vi "Filter Out Combined Source.vi"(1 "Sources In":T1[](array[typedef])) -> (0 "Sources Out":T1[](array[typedef]))   [LabVIEW 2009]
uses:
  Global Data/Transactions/Dataset Source.ctl
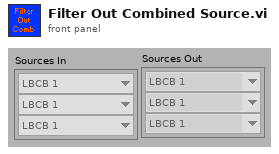
[diagram p1: front panel]
types:
  T1 = typedef "Dataset Source.ctl" = enum16{"LBCB 1", "LBCB 2", "Combined", "External Sensors"}
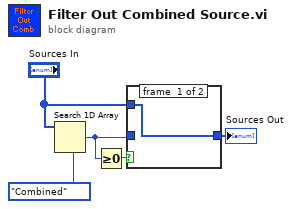
[diagram p0: block diagram]
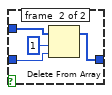
[diagram p2: hidden frame]
diagram:
  n1 = Search 1D Array(1D array="Sources In", element=Dataset_Source."Combined") -> (index of element=w5:i32)  [unwired: 1 in]
  n2 = Greater Or Equal To 0?(x=w5) -> (x >= 0?=w4:bool)
  n3 = case shown="False" w4 {
    tunnel: "Sources In" -> [w6 w10]
    tunnel: w5 -> [_ w8]
    tunnel: [w6 w7] -> w3
    frame #0 {
    }
    frame #1 {
      n4 = Delete From Array(array=w10, length=1, index=w8) -> (array with subset deleted=w7:T1[])  [unwired: 1 out]
    }
  }
  "Sources Out" <- w3
